vi "ActivateProvider.vi"   [LabVIEW 2016]
types:
  T1 = enum16{"Left Button", "Center Button", "Right Button", "Window Close"}
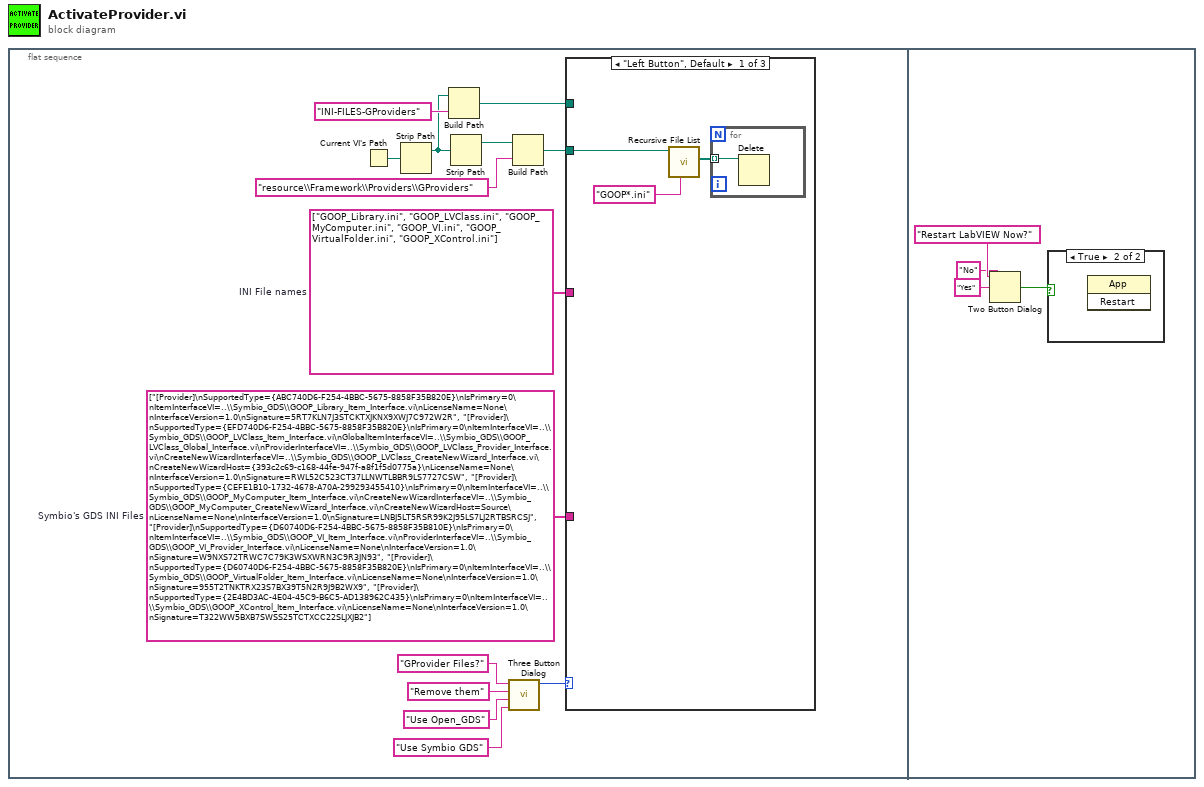
[diagram p0: block diagram]
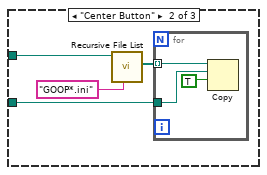
[diagram p2: hidden frame]
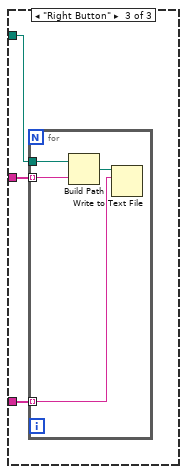
[diagram p3: hidden frame]
diagram:
  n1 = flat-sequence {
    frame #0 {
      w2 = string[] ["GOOP_Library.ini", "GOOP_LVClass.ini", "GOOP_MyComputer.ini", "GOOP_VI.ini", "GOOP_VirtualFolder.ini", "GOOP_XControl.ini"]  # INI File names
      w1 = string[] ["[Provider]\nSupportedType={ABC740D6-F254-4BBC-5675-8858F35B820E}\nIsPrimary=0\nItemInterfaceVI=..\\Symbio_GDS\\GOOP_Library_Item_Interface.vi\nLicenseName=None\nInterfaceVersion=1.0\nSignature=5RT7KLN7J3STCKTXJKNX9XWJ7C972W2R", "[Provider]\nSupportedType={EFD740D6-F254-4BBC-5675-8858F35B820E}\nIsPrimary=0\nItemInterfaceVI=..\\Symbio_GDS\\GOOP_LVClass_Item_Interface.vi\nGlobalItemInterfaceVI=..\\Symbio_GDS\\GOOP_LVClass_Global_Interface.vi\nProviderInterfaceVI=..\\Symbio_GDS\\GOOP_LVClass_Provider_Interface.vi\nCreateNewWizardInterfaceVI=..\\Symbio_GDS\\GOOP_LVClass_CreateNewWizard_Interface.vi\nCreateNewWizardHost={393c2c69-c168-44fe-947f-a8f1f5d0775a}\nLicenseName=None\nInterfaceVersion=1.0\nSignature=RWL52C523CT37LLNWTLBBR9LS7727CSW", "[Provider]\nSupportedType={CEFE1B10-1732-4678-A70A-299293455410}\nIsPrimary=0\nItemInterfaceVI=..\\Symbio_GDS\\GOOP_MyComputer_Item_Interface.vi\nCreateNewWizardInterfaceVI=..\\Symbio_GDS\\GOOP_MyComputer_CreateNewWizard_Interface.vi\nCreateNewWizardHost=Source\nLicenseName=None\nInterfaceVersion=1.0\nSignature=LNBJ5LT5RSR99K2J95LS7LJ2RTBSRCSJ", "[Provider]\nSupportedType={D60740D6-F254-4BBC-5675-8858F35B810E}\nIsPrimary=0\nItemInterfaceVI=..\\Symbio_GDS\\GOOP_VI_Item_Interface.vi\nProviderInterfaceVI=..\\Symbio_GDS\\GOOP_VI_Provider_Interface.vi\nLicenseName=None\nInterfaceVersion=1.0\nSignature=W9NXS72TRWC7C79K3WSXWRN3C9R3JN93", "[Provider]\nSupportedType={D60740D6-F254-4BBC-5675-8858F35B820E}\nIsPrimary=0\nItemInterfaceVI=..\\Symbio_GDS\\GOOP_VirtualFolder_Item_Interface.vi\nLicenseName=None\nInterfaceVersion=1.0\nSignature=955T2TNKTRX23S7BX39T5N2R9J9B2WX9", "[Provider]\nSupportedType={2E4BD3AC-4E04-45C9-B6C5-AD138962C435}\nIsPrimary=0\nItemInterfaceVI=..\\Symbio_GDS\\GOOP_XControl_Item_Interface.vi\nLicenseName=None\nInterfaceVersion=1.0\nSignature=T322WW5BXB7SWSS25TCTXCC22SLJXJB2"]  # Symbio's GDS INI Files
      n2 = Current VI's Path() -> (path=w5:path)
      n3 = Strip Path(path=w5) -> (stripped path=w4:path)  [unwired: 1 out]
      n4 = Build Path(base path=w4, name or relative path="INI-FILES-GProviders") -> (appended path=w3:path)
      n5 = Strip Path(path=w4) -> (stripped path=w8:path)  [unwired: 1 out]
      n6 = call <vilib>:"Three Button Dialog.vi"("Right Button Text (\"Cancel\")"="Use Symbio GDS" ("Right Button Text (\"Cancel\")"), "Center Button Text (\"No\")"="Use Open_GDS" ("Center Button Text (\"No\")"), "Left Button Text (\"Yes\")"="Remove them" ("Left Button Text (\"Yes\")"), "message"="GProvider Files?") -> ("Which Button?"=w10:T1)  [unwired: 7 in]
      n7 = Build Path(base path=w8, name or relative path="resource\\Framework\\Providers\\GProviders") -> (appended path=w7:path)
      n8 = case shown="\"Left Button\", Default" w10 {
        tunnel: w7 -> [w16 w20 w28]
        tunnel: w3 -> [_ w22 _]
        tunnel: w2 -> [_ _ w27]
        tunnel: w1 -> [_ _ w26]
        frame "Left Button", Default {
          n9 = call <vilib>:"Recursive File List.vi"("pattern"="GOOP*.ini", "Folder Path"=w16) -> ("All Files in Dir"=w15:path[])  [unwired: 5 in, 4 out]
          n10 = for {
            tunnel: w15 -> [w18] mode=indexing
            n11 = Delete(path (use dialog)=w18) -> ()  [unwired: 4 in, 3 out]
          }
        }
        frame "Center Button" {
          n12 = call <vilib>:"Recursive File List.vi"("pattern"="GOOP*.ini", "Folder Path"=w22) -> ("All Files in Dir"=w21:path[])  [unwired: 5 in, 4 out]
          n13 = for {
            tunnel: w21 -> [w25] mode=indexing
            tunnel: w20 -> [w24]
            n14 = Copy(9:TRUE ("overwrite (F)"), 10:w24, 11:w25) -> ()  [unwired: 2 in, 3 out]
          }
        }
        frame "Right Button" {
          n15 = for {
            tunnel: w28 -> [w32]
            tunnel: w27 -> [w30] mode=indexing
            tunnel: w26 -> [w29] mode=indexing
            n16 = Build Path(base path=w32, name or relative path=w30) -> (appended path=w31:path)
            n17 = Write to Text File(file (use dialog)=w31, text=w29) -> ()  [unwired: 2 in, 3 out]
          }
        }
      }
    }
    frame #1 {
      n18 = Two Button Dialog(message="Restart LabVIEW Now?", 1:"No" ("F button name (\"Cancel\")"), 2:"Yes" ("T button name (\"OK\")")) -> (T button?=w33:bool)
      n19 = case shown="True" w33 {
        frame False {
        }
        frame True {
          n20 = invoke class="App" method="Restart"() -> ()  [unwired: 3 in, 3 out]
        }
      }
    }
  }
